vi "read config.vi"(8 "error in (no error)":errorcluster, 10 "File Path":path, 11 "Wheatstone Bridge in":refnum<class "Wheatstone Bridge.lvclass">) -> (0 "error out":errorcluster, 3 "Wheatstone Bridge out":refnum<class "Wheatstone Bridge.lvclass">)   [LabVIEW 2025, in "Wheatstone Bridge.lvlib" / "Wheatstone Bridge.lvclass"]
uses:
  Wheatstone Bridge.lvclass
  Wheatstone Bridge.lvclass/Wheatstone Bridge.ctl
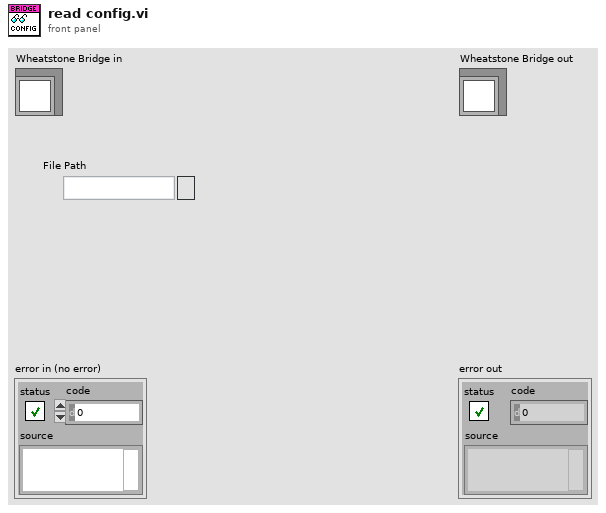
[diagram p1: front panel]
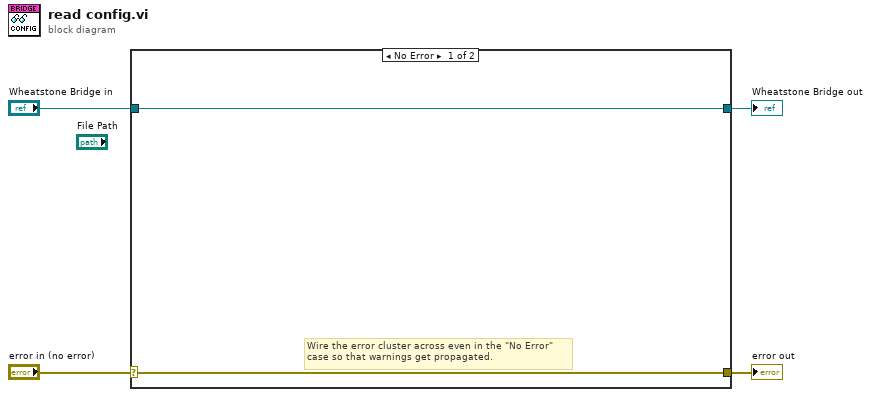
[diagram p0: block diagram]
diagram:
  n1 = case shown="No Error" "error in (no error)" {
    selector: "error in (no error)" -> [w5 w8]
    tunnel: [w5 w8] -> w3
    tunnel: [w6 w7] -> w1
    tunnel: "Wheatstone Bridge in" -> [w6 w7]
    frame No Error {
      # "Wire the error cluster across even in the \"No Error\"\ncase so that warnings get propagated."
    }
    frame Error {
    }
  }
  "error out" <- w3
  "Wheatstone Bridge out" <- w1
